vi "Mem_U32Array.vi"(8 "error in (no error)":errorcluster, 11 "dataInfo":T1) -> (0 "error out":errorcluster, 2 "DataPoints":u32[](array[numeric]))   [LabVIEW 2019, in "Memory Data Access.lvlib"]
uses:
  Memory Data Access.lvlib
  Typedef/memoryDataBlock.ctl
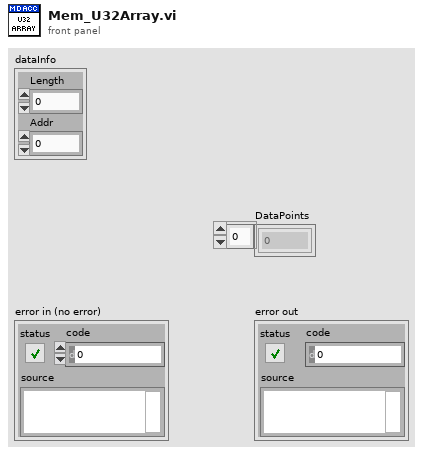
[diagram p1: front panel]
types:
  T1 = typedef "Memory Data Access.lvlib/memoryDataBlock.ctl" = cluster{"Length":u32, "Addr":u64}
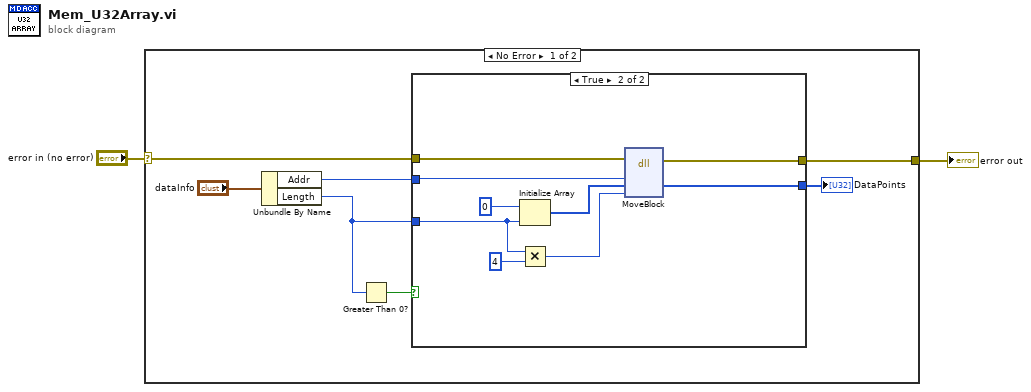
[diagram p0: block diagram]
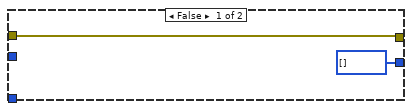
[diagram p2: hidden frame]
diagram:
  n1 = case shown="No Error" "error in (no error)" {
    selector: "error in (no error)" -> [w9 w21]
    tunnel: [w8 w21] -> w1
    frame No Error {
      n2 = Unbundle By Name("dataInfo") -> ("Addr"=w4:u64, "Length"=w3:u32)
      n3 = Greater Than 0?(x=w3) -> (x > 0?=w7:bool)
      n4 = case shown="True" w7 {
        tunnel: w9 -> [w11 w20]
        tunnel: [w11 w19] -> w8
        tunnel: w4 -> [_ w13]
        tunnel: w3 -> [_ w14]
        tunnel: [u32[] [] ("Destination") w12] -> w6
        frame False {
        }
        frame True {
          n5 = Initialize Array(u32 0, w14) -> (w17:u32[])
          n6 = Multiply(x=w14, y=u32 4) -> (x*y=w15:u32)
          n7 = dll-call lib="LabVIEW" fn="MoveBlock"(error in=w20, "Address"=w13, "Destination"=w17, "Size"=w15) -> (error out=w19:errorcluster, "Destination"=w12:u32[])  [unwired: 5 in, 1 out]
        }
      }
      "DataPoints" <- w6
    }
    frame Error {
    }
  }
  "error out" <- w1
